vi "RT_Test_DAQmx.vi"() -> ()   [LabVIEW 2020]
uses:
  <vilib>/DAQmx/read.llb/DAQmx Read (Analog 1D Wfm NChan NSamp).vi
  <vilib>/DAQmx/create/channels.llb/DAQmx Create Channel (AI-Voltage-Basic).vi
  <vilib>/DAQmx/configure/timing.llb/DAQmx Timing (Sample Clock).vi
  <vilib>/DAQmx/miscellaneous.llb/DAQmx Fill In Error Info.vi
  <resource>/objmgr/daqmx.rc
panel:
  in  "error in":errorcluster
  out "data":waveform(dbl)(graph)
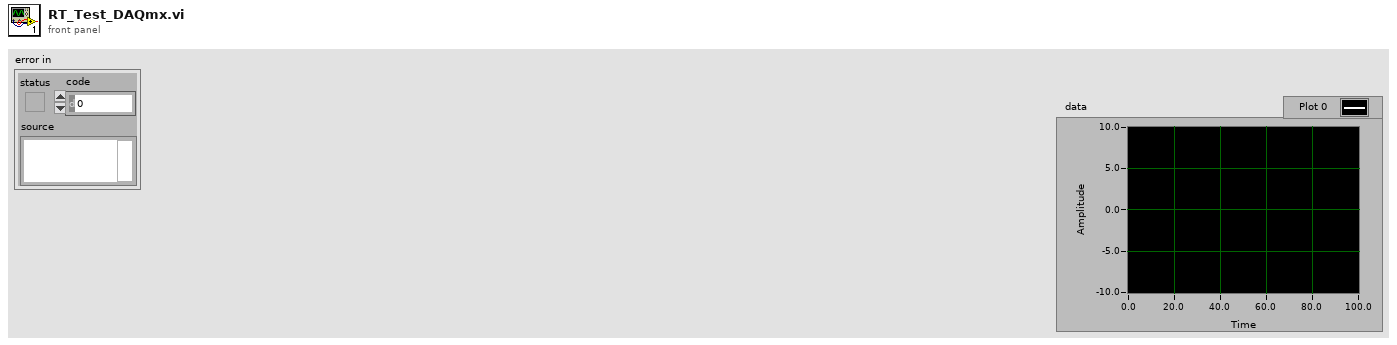
[diagram p1: front panel]
types:
  T1 = enum16{"open", "open or create", "create or replace", "create", "open (read-only)"}
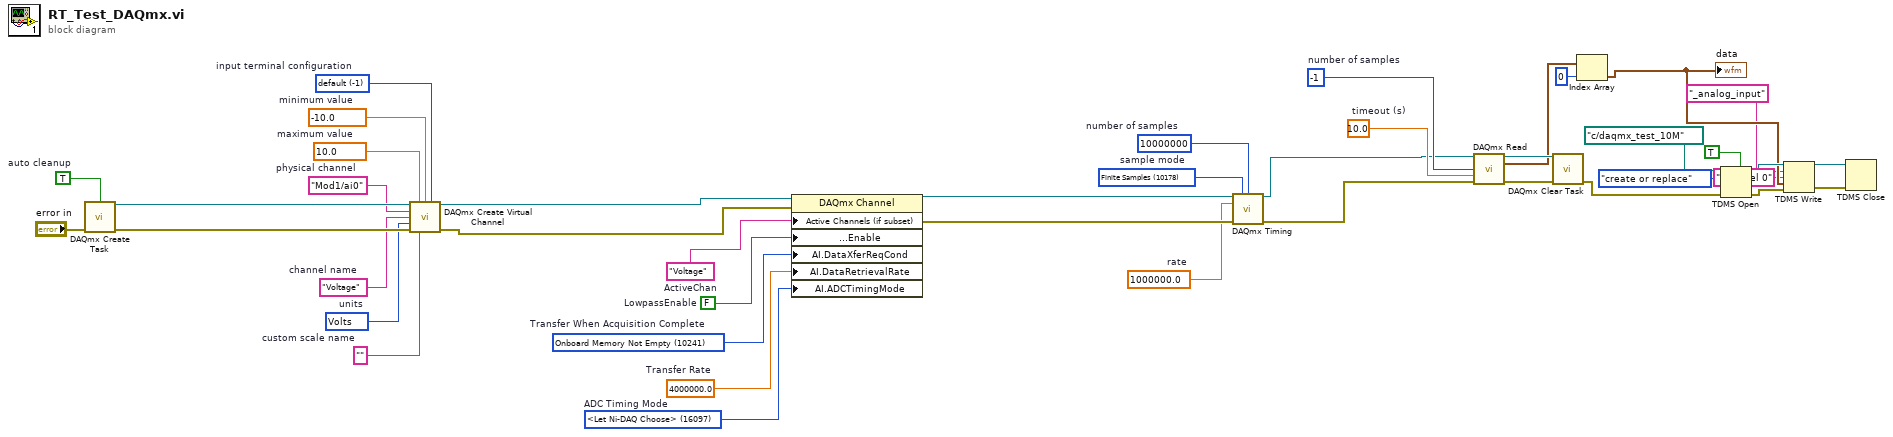
[diagram p0: block diagram]
diagram:
  w16 = 10178 items=["Finite Samples"=10178, "Continuous Samples"=10123, "Hardware Timed Single Point"=12522]  # sample mode
  w17 = 10000000  # number of samples
  w18 = 1000000.0  # rate
  w20 = 4000000.0  # Transfer Rate
  w21 = 16097 items=["<Let Ni-DAQ Choose>"=16097, "High Resolution"=10195, "High Speed"=14712]  # ADC Timing Mode
  w22 = 10241 items=["Onboard Memory More than Half Full"=10237, "Onboard Memory Not Empty"=10241, "Onboard Memory Custom Threshold"=12577, "When Acquisition Complete"=12546]  # Transfer When Acquisition Complete
  w24 = FALSE  # LowpassEnable
  w26 = "Voltage"  # ActiveChan
  w27 = -1 items=["default"=-1, "RSE"=10083, "NRSE"=10078, "Differential"=10106, "Pseudodifferential"=12529]  # input terminal configuration
  w28 = 10348 items=["Volts"=10348, "From Custom Scale"=10065]  # units
  w29 = "Voltage"  # channel name
  w31 = ""  # custom scale name
  w32 = -10.0  # minimum value
  w33 = 10.0  # maximum value
  w34 = "Mod1/ai0"  # physical channel
  w36 = TRUE  # auto cleanup
  w41 = 10.0  # timeout (s)
  w42 = -1  # number of samples
  n1 = call <vilib>:"DAQmx Create Task.vi"("auto cleanup"=w36, "error in"="error in") -> ("task out"=w35:refnum<k21>, "error out"=w37:errorcluster)  [unwired: 12 in]
  n2 = call-poly <vilib>:"DAQmx Create Virtual Channel.vi"("task in"=w35, "maximum value"=w33, "minimum value"=w32, "input terminal configuration"=w27, "physical channels"=w34, "name to assign"=w29, "units"=w28, "error in"=w37, "custom scale name"=w31) -> ("task out"=w23:refnum<k21>, "error out"=w30:errorcluster)  [unwired: 5 in]
  n3 = property class="DAQmx Channel"(reference=w23, error in=w30, "Active Channels (if subset)"=w26, "Analog Input:General Properties:Filter:Analog Lowpass:Enable"=w24, "AI.DataXferReqCond"=w22, "AI.DataRetrievalRate"=w20, "AI.ADCTimingMode"=w21) -> (reference out=w19:refnum<k21>, error out=w25:errorcluster)
  n4 = call-poly <vilib>:"DAQmx Timing.vi"("task/channels in"=w19, "sample mode"=w16, "samples per channel"=w17, "rate"=w18, "error in"=w25) -> ("task out"=w15:refnum<k21>, "error out"=w14:errorcluster)  [unwired: 9 in]
  n5 = call-poly <vilib>:"DAQmx Read.vi"("task/channels in"=w15, "number of samples per channel"=w42, "timeout"=w41, "error in"=w14) -> ("task out"=w39:refnum<k21>, "data"=w13:waveform(dbl)[], "error out"=w40:errorcluster)  [unwired: 9 in]
  n6 = call <vilib>:"DAQmx Clear Task.vi"("task in"=w39, "error in"=w40) -> ("error out"=w9:errorcluster)  [unwired: 13 in]
  n7 = Index Array(array=w13, index=0) -> (element=w5:waveform(dbl))
  "data" <- w5
  n8 = TDMS Open(5:TRUE ("create index file? (T)"), 8:w9, 10:T1."create or replace" ("operation (0:open)"), 11:path "c:/daqmx_test_10M" ("file path")) -> (0:w6:errorcluster, 3:w7:refnum<k34>)  [unwired: 3 in]
  n9 = TDMS Write(0:w7, 5:"_analog_input" ("group name in (Untitled)"), 7:"Channel 0" ("channel name(s) in (Untitled)"), 9:w5, 11:w6) -> (4:w2:refnum<k34>, 15:w1:errorcluster)  [unwired: 1 in, 2 out]
  n10 = TDMS Close(8:w1, 11:w2) -> ()  [unwired: 2 out]
